vi "MEMR-Compute Metrics.vi"(0 "Gain spectra in":cluster{"Freq (Hz)":dbl[], "Mag":dbl[][]}[](array[cluster]), 5 "Compute":enum16{"Mean", "Sum"}(ring), 7 "Scale":enum16{"Linear", "Log"}(ring), 9 "Fpeak":dbl[](array[numeric]), 11 "Measure":T1(ring)) -> (4 "Gain spectra out":cluster{"Freq (Hz)":dbl[], "Mag":dbl[][]}[](array[cluster]), 8 "Metrics":dbl[][](array[numeric]))   [LabVIEW 2020]
uses:
  <vilib>/Analysis/baseanly.llb/Mean (DBL).vi
  Utility VIs/Math VIs/interp1 (1D).vi
  Utility VIs/Array Manipulation VIs/Irregular Array Subset (DBL).vi
  Utility VIs/Math VIs/dB to Linear (1D).vi
  Utility VIs/Math VIs/Linear to dB (scalar).vi
  <vilib>/Analysis/NI_AALBase.lvlib
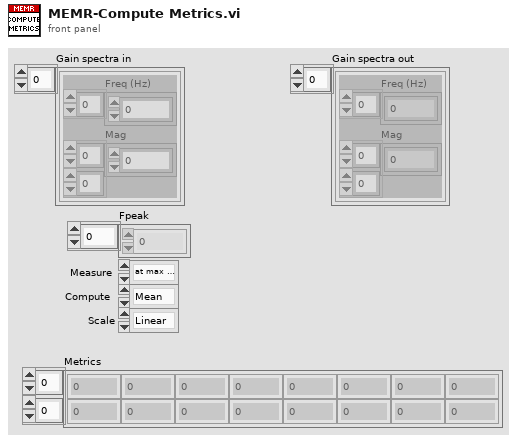
[diagram p1: front panel]
types:
  T1 = enum16{"at max mag", "at max gain", "over window", "optimize", "Keefe"}
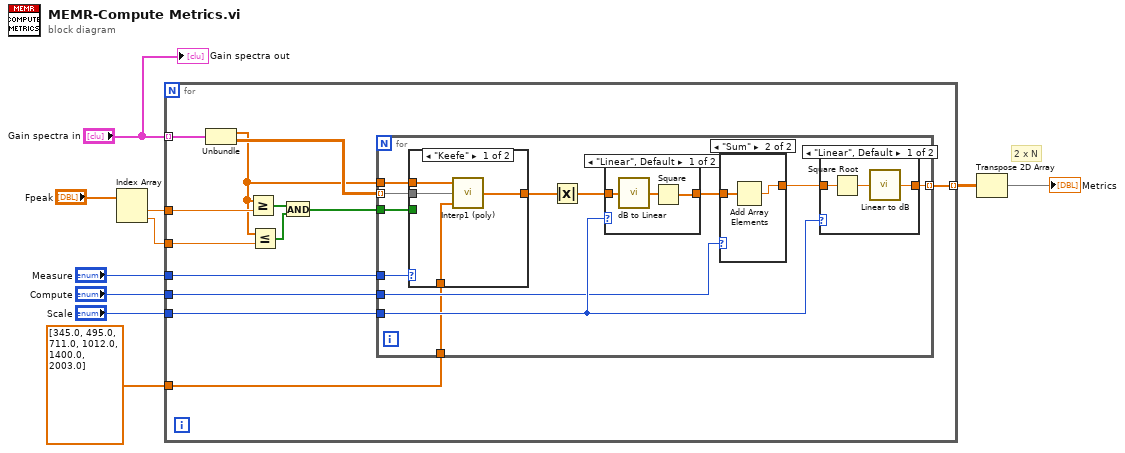
[diagram p0: block diagram]
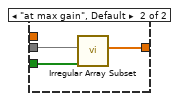
[diagram p2: hidden frame]
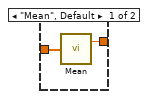
[diagram p3: hidden frame]
diagram:
  # "2 x N"
  n1 = Index Array(array="Fpeak") -> (element #1=w6:dbl, element #2=w5:dbl)  [unwired: 2 in]
  n2 = for {
    tunnel: "Gain spectra in" -> [w23] mode=indexing
    tunnel: [w22] -> w9 mode=indexing
    tunnel: w6 -> [w17]
    tunnel: w5 -> [w16]
    tunnel: "Scale" -> [w15]
    tunnel: "Compute" -> [w14]
    tunnel: "Measure" -> [w13]
    tunnel: dbl[] [345.0, 495.0, 711.0, 1012.0, 1400.0, 2003.0] -> [w11]
    n3 = Unbundle(w23) -> ("Freq (Hz)"=w12:dbl[], "Mag"=w18:dbl[][])
    n4 = Greater Or Equal?(x=w12, y=w17) -> (x >= y?=w19:bool[])
    n5 = Less Or Equal?(x=w12, y=w16) -> (x <= y?=w20:bool[])
    n6 = And(x=w19, y=w20) -> (x .and. y?=w21:bool[])
    n7 = for {
      tunnel: w21 -> [w34]
      tunnel: w18 -> [w33] mode=indexing
      tunnel: [w32] -> w22 mode=indexing
      tunnel: w15 -> [w28]
      tunnel: w14 -> [w27]
      tunnel: w13 -> [w26]
      tunnel: w12 -> [w25]
      tunnel: w11 -> [w24]
      n8 = case shown="\"Keefe\"" w26 {
        tunnel: [w37 w42] -> w35
        tunnel: w34 -> [_ w41]
        tunnel: w33 -> [w39 w40]
        tunnel: w25 -> [w38 _]
        tunnel: w24 -> [w36 _]
        frame "Keefe" {
          n9 = call-poly "Interp1 (poly).vi"("X"=w38, "Y"=w39, "U"=w36) -> ("V"=w37:dbl[])  [unwired: 2 in]
        }
        frame "at max gain", Default {
          n10 = call-poly "Irregular Array Subset.vi"("Mask"=w41, "Array"=w40) -> ("Array Subset"=w42:dbl[])  [unwired: 8 in, 1 out]
        }
      }
      n11 = Absolute Value(x=w35) -> (abs(x)=w29:dbl[])
      n12 = case shown="\"Linear\", Default" w28 {
        tunnel: [w49 w50] -> w30
        tunnel: w29 -> [w48 w50]
        frame "Linear", Default {
          n13 = call-poly "dB to Linear.vi"("dB"=w48) -> ("linear"=w47:dbl[])
          n14 = Square(x=w47) -> (x^2=w49:dbl[])
        }
        frame "Log" {
        }
      }
      n15 = case shown="\"Sum\"" w27 {
        tunnel: [w44 w46] -> w31
        tunnel: w30 -> [w43 w45]
        frame "Mean", Default {
          n16 = call-poly <vilib>:"Mean.vi"("X"=w43) -> ("mean"=w44:dbl)  [unwired: 1 out]
        }
        frame "Sum" {
          n17 = Add Array Elements(numeric array=w45) -> (sum=w46:dbl)
        }
      }
      n18 = case shown="\"Linear\", Default" w28 {
        tunnel: [w53 w54] -> w32
        tunnel: w31 -> [w51 w54]
        frame "Linear", Default {
          n19 = Square Root(x=w51) -> (sqrt(x)=w52:dbl)
          n20 = call-poly "Linear to dB.vi"("Linear"=w52) -> ("dB"=w53:dbl)
        }
        frame "Log" {
        }
      }
    }
  }
  n21 = Transpose 2D Array(2D array=w9) -> (transposed array=→"Metrics":dbl[][])
  "Gain spectra out" <- "Gain spectra in"
